vi "solar_excel Workbook Create.vi"(8 "error in (no error)":errorcluster, 10 "Worksheet":string, 11 "Excel App":T1) -> (0 "error out":errorcluster, 3 "Excel Workbook":T2)   [LabVIEW 2018]
doc: "This creates a new Workbook with one <b>Worksheet</b> and returns the Workbook reference."
uses:
  solar_excel_ctl Workbook.ctl
  solar_excel_ctl TSV.ctl
  solar_excel_ctl App.ctl
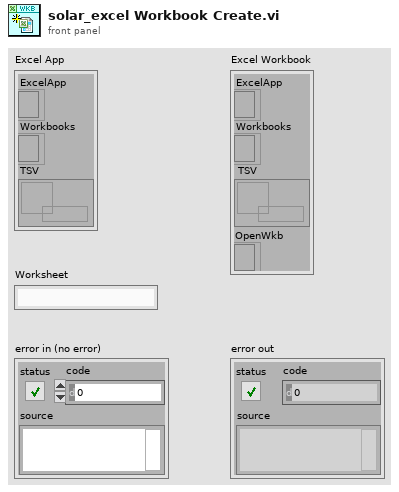
[diagram p1: front panel]
types:
  T1 = typedef "solar_excel_ctl App.ctl" = cluster{"ExcelApp":refnum<k7>, "Workbooks":refnum<k7>, "TSV":refnum<queue>}
  T2 = typedef "solar_excel_ctl Workbook.ctl" = cluster{"ExcelApp":refnum<k7>, "Workbooks":refnum<k7>, "TSV":refnum<queue>, "OpenWkb":refnum<k7>}
  T3 = typedef "solar_excel_ctl TSV.ctl" = cluster{"Path":path, "Dirty":bool, "ActiveSheet":u8, "Worksheets":string[], "Worksheet Cells":cluster{"Cells":string[][]}[]}
  T4 = typedef "solar_excel_ctl Worksheet.ctl" = cluster{"ExcelApp":refnum<k7>, "Workbooks":refnum<k7>, "TSV":refnum<queue>, "OpenWkb":refnum<k7>, "Worksheets":refnum<k7>, "OpenWksh":refnum<k7>}
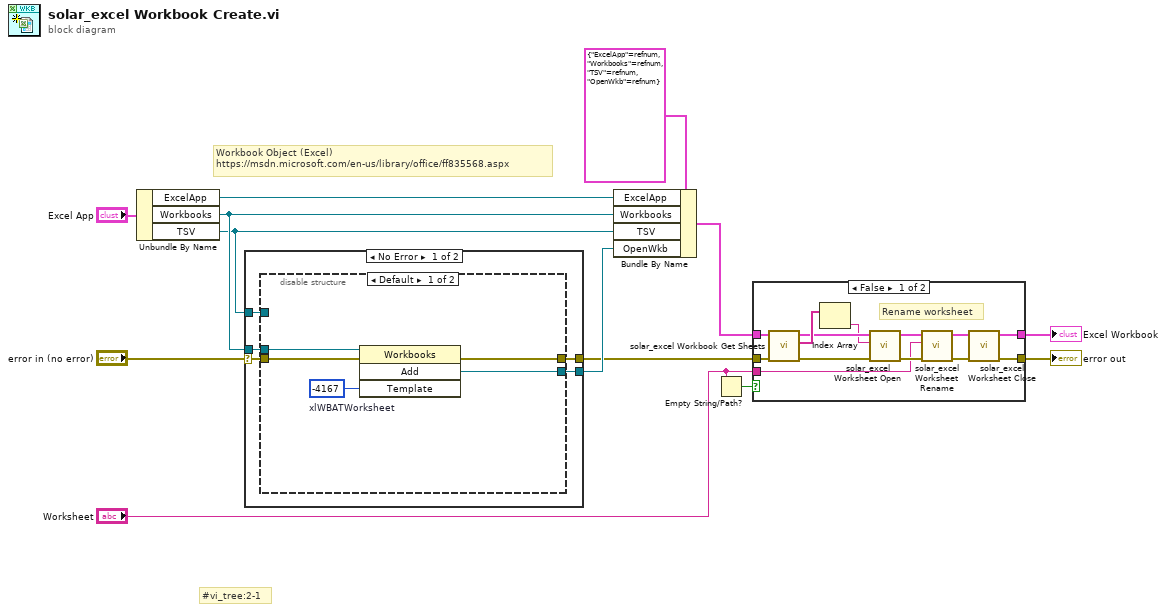
[diagram p0: block diagram]
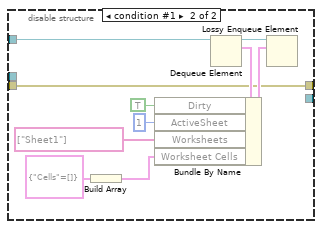
[diagram p3: hidden frame]
diagram:
  # "#vi_tree:2-1"
  # "Workbook Object (Excel)\nhttps://msdn.microsoft.com/en-us/library/office/ff835568.aspx"
  n1 = Unbundle By Name("Excel App") -> ("ExcelApp"=w10:refnum<k7>, "Workbooks"=w9:refnum<k7>, "TSV"=w1:refnum<queue>)
  n2 = case shown="No Error" "error in (no error)" {
    selector: "error in (no error)" -> [w18 w34]
    tunnel: [w16 w34] -> w6
    tunnel: w9 -> [w17 _]
    tunnel: [w15 _] -> w8
    tunnel: w1 -> [w14 _]
    frame No Error {
      n3 = disable-structure shown="Default" {
        disable-tunnel: w18 -> [w23 w29]
        disable-tunnel: w17 -> [w22 _]
        disable-tunnel: [w20 w29] -> w16
        disable-tunnel: [w19 _] -> w15
        disable-tunnel: w14 -> [_ w33]
        frame condition #0 (active) {
          w21 = -4167  # xlWBATWorksheet
          n4 = invoke class="Workbooks" method="Add"(reference=w22, error in=w23, "Template"=w21) -> (error out=w20:errorcluster, "Add"=w19:refnum<k7>)  [unwired: 1 in, 2 out]
        }
        frame condition #1 {
          n5 = Build Array(cluster{"Cells":string[][]} {"Cells"=[]} ("Worksheet Data")) -> (w24:cluster{"Cells":string[][]}[])
          n6 = Dequeue Element(queue=w33) -> (queue out=w32:refnum<queue>, element=w31:T3)  [unwired: 2 in, 2 out]
          n7 = Bundle By Name(cluster=w31, "Dirty"=TRUE, "ActiveSheet"=u8 1, "Worksheets"=string[] ["Sheet1"], "Worksheet Cells"=w24) -> (w30:T3)
          n8 = Lossy Enqueue Element(queue=w32, element=w30) -> ()  [unwired: 1 in, 4 out]
        }
      }
    }
    frame Error {
    }
  }
  n9 = Bundle By Name(cluster=T2 {"ExcelApp"=refnum, "Workbooks"=refnum, "TSV"=refnum, "OpenWkb"=refnum} ("Excel Workbook"), "ExcelApp"=w10, "Workbooks"=w9, "TSV"=w1, "OpenWkb"=w8) -> (w5:T2)
  n10 = Empty String/Path?(string/path="Worksheet") -> (empty?=w2:bool)
  n11 = case shown="False" w2 {
    tunnel: "Worksheet" -> [w39 _]
    tunnel: [w38 w49] -> w7
    tunnel: w6 -> [w37 w49]
    tunnel: w5 -> [w36 w48]
    tunnel: [w35 w48] -> w4
    frame False {
      # "Rename worksheet"
      n12 = call "solar_excel Workbook Get Sheets.vi"("error in (no error)"=w37, "Excel Workbook in"=w36) -> ("error out"=w46:errorcluster, "Worksheet Names"=w47:string[], "Excel Workbook out"=w45:T2)  [unwired: 6 in, 1 out]
      n13 = Index Array(array=w47) -> (element=w44:string)  [unwired: 1 in]
      n14 = call "solar_excel Worksheet Open.vi"("error in (no error)"=w46, "Sheet Name (STR) or Number (I32)"=w44, "Excel Workbook"=w45) -> ("error out"=w43:errorcluster, "Excel Worksheet"=w42:T4)  [unwired: 5 in, 2 out]
      n15 = call "solar_excel Worksheet Rename.vi"("error in (no error)"=w43, "New Worksheet Name"=w39, "Excel Worksheet in"=w42) -> ("error out"=w41:errorcluster, "Excel Worksheet out"=w40:T4)  [unwired: 7 in]
      n16 = call "solar_excel Worksheet Close.vi"("error in (no error)"=w41, "Excel Worksheet"=w40) -> ("error out"=w38:errorcluster, "Excel Workbook"=w35:T2)  [unwired: 8 in]
    }
    frame True {
    }
  }
  "error out" <- w7
  "Excel Workbook" <- w4
